vi "Arm Controller.vi"(8 "error in":errorcluster) -> ()   [LabVIEW 2017]
doc: "This VI executes continuously carrying out the current operation and responding to updates or new operations. It will often contain the timing or control code that is difficult to place directly in TeleOp. This VI generally opens all sensors and motors and isolates the rest of the robot code from knowing how the operations are carried out."
uses:
  <vilib>/Rock Robotics/WPI/Framework/Completion Status.ctl
  Arm Setpoints.ctl
  Arm Operations.ctl
  <vilib>/Rock Robotics/SystemInterfaces/DIO/FPGA_DIOPWMChannel.ctl
  <vilib>/Rock Robotics/SystemInterfaces/DIO/FPGA_DIOChannel.ctl
  <vilib>/Rock Robotics/WPI/Switch/WPI_SwitchOpenLimit.vi
  <vilib>/Rock Robotics/WPI/MotorControl/WPI_MotorControlOpen SPARK.vi
  Framework/Robot Global Data.vi
  <vilib>/Rock Robotics/Network Tables/NT Write Number.vi
panel:
  out "Lower Arm Limit Switch":bool
  out "Lift Arm Limit Switch":bool
  out "Switch Value":bool
  in  "Interactive Values":T1
  out "Current\nCmd":string
  in  "Buttons":cluster{"Execute Cmd":bool, "Abort Cmd":bool}
  out "Command Timing":cluster{"Start Time (ms)":u32, "Iterations":i32}
  out "Status":T3
  # "Tip: It may be helpful to observe inputs and sensor values.\nYou may also want to display tuning or debugging controls."
  # "Interactive Command: You may fill in the settings for a command\nand schedule it with the Execute button. You can observe and abort\nany command while fine tuning the code for the controller."
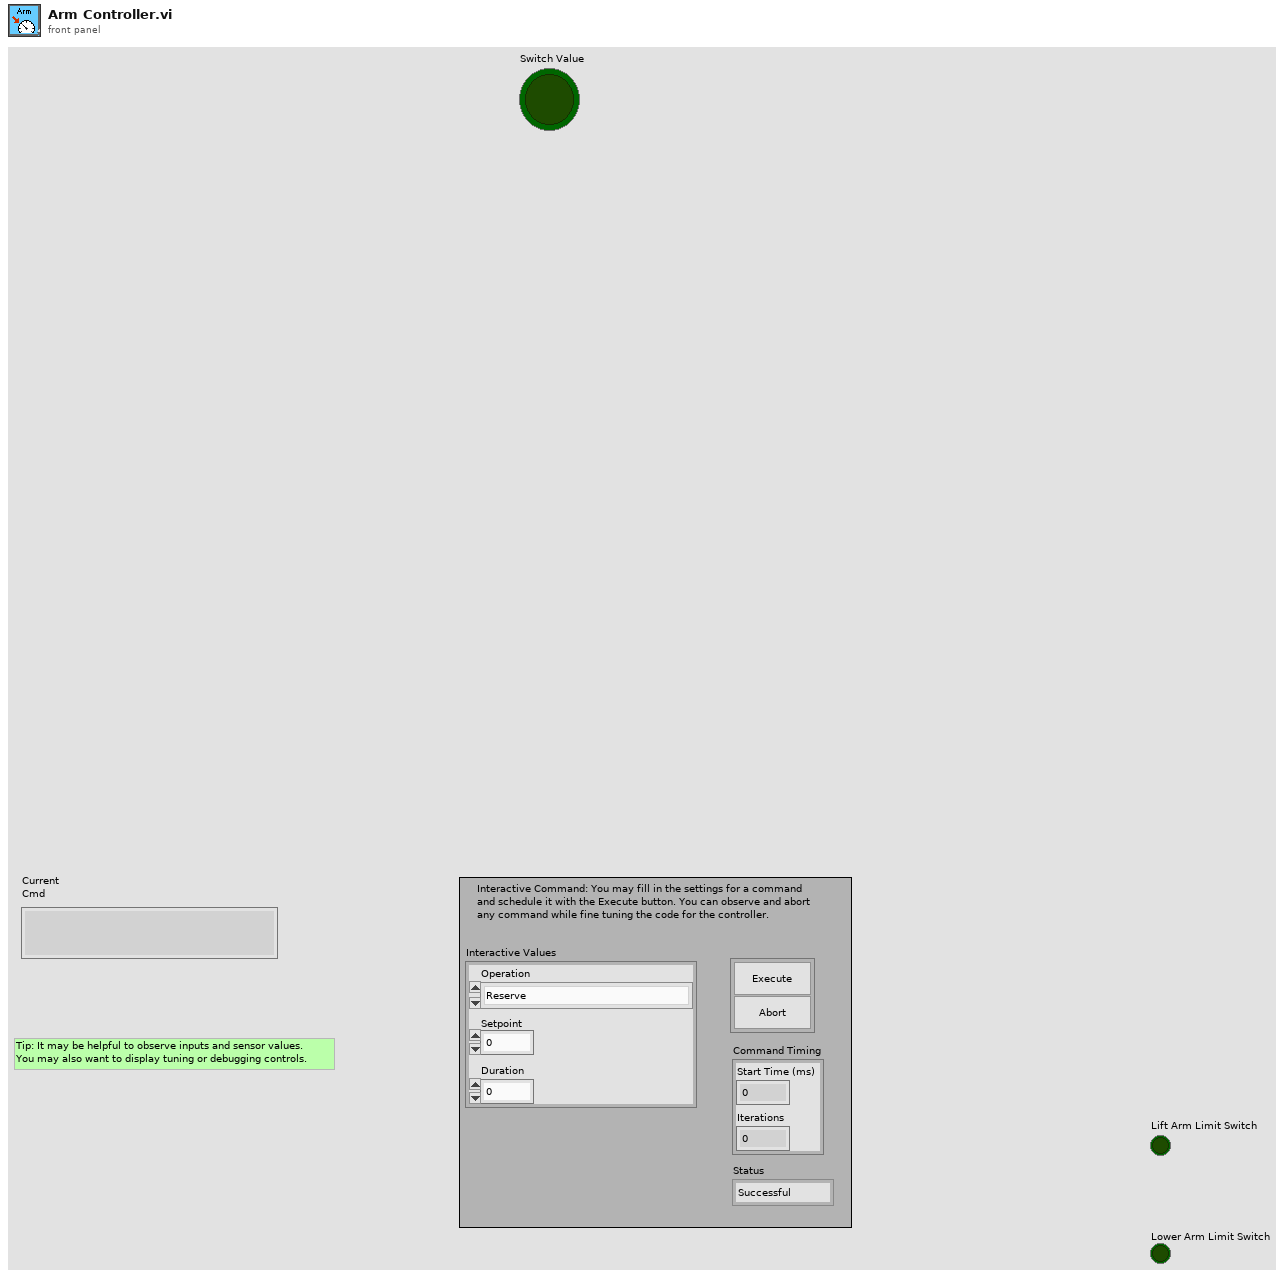
[diagram p1: front panel]
types:
  T1 = typedef "Arm Setpoints.ctl" = cluster{"Operation":T2, "Setpoint":dbl, "Duration":dbl}
  T2 = typedef "Arm Operations.ctl" = enum16{"Reserve", "Read Current", "Immediate", "Lift Arm", "Lower Arm ", "Button Lift Arm", "Button Lower Arm"}
  T3 = typedef "Completion Status.ctl" = enum16{"Successful", "Aborted", "Incomplete"}
  T4 = typedef "FPGA_DIOChannel.ctl" = enum8{"DIO 0", "DIO 1", "DIO 2", "DIO 3", "DIO 4", "DIO 5", "DIO 6", "DIO 7", "DIO 8", "DIO 9", "DIO MXP 0", "DIO MXP 1", "DIO MXP 2", "DIO MXP 3", "DIO MXP 4", "DIO MXP 5", "DIO MXP 6", "DIO MXP 7", "DIO MXP 8", "DIO MXP 9", "DIO MXP 10", "DIO MXP 11", "DIO MXP 12", "DIO MXP 13", "DIO MXP 14", "DIO MXP 15", "SPI Port CS1", "SPI Port CS2", "SPI Port CS3", "SPI Port MISO", "SPI Port MOSI", "Invalid"}
  T5 = typedef "FPGA_DIOPWMChannel.ctl" = enum8{"PWM 0", "PWM 1", "PWM 2", "PWM 3", "PWM 4", "PWM 5", "PWM 6", "PWM 7", "PWM 8", "PWM 9", "PWM MXP 0", "PWM MXP 1", "PWM MXP 2", "PWM MXP 3", "PWM MXP 4", "PWM MXP 5", "PWM MXP 6", "PWM MXP 7", "PWM MXP 8", "PWM MXP 9", "Invalid"}
  T6 = typedef "WPI_MotorControlDeviceRef.ctl" = cluster{"DeviceStatus":errorcluster, "Type":T7, "PWM":cluster{"PWM Channel":T5, "DeadBand":T8}, "CAN":cluster{"Device Number":u8, "SetOutput VI Ref":variant, "GetOutput VI Ref":variant, "Enable VI Ref":variant, "Disable VI Ref":variant, "Data":variant}, "Invert":bool, "DIO PWM":cluster{"PWM \"Enable\" Channel":T5, "DIOChannel":T4, "PWM Rate":dbl}}
  T7 = typedef "WPI_MotorControlType.ctl" = enum16{"PWM", "CAN", "DIO PWM"}
  T8 = typedef "WPI_PWMDeadband.ctl" = cluster{"Name":string, "maxPositivePwm":i32, "minPositivePwm":i32, "centerPwm":i32, "maxNegativePwm":i32, "minNegativePwm":i32, "angularRange":u16}
  T9 = typedef "WPI_SwitchDevRef.ctl" = cluster{"DevStatus":errorcluster, "DIO Channel":T4, "CntIndex":T10, "Normally Closed":bool}
  T10 = typedef "FPGA_CounterCtrSystemIndex.ctl" = enum8{"Ctr 0", "Ctr 1", "Ctr 2", "Ctr 3", "Ctr 4", "Ctr 5", "Ctr 6", "Ctr 7", "Invalid"}
  T11 = typedef "Command Status Info.ctl" = cluster{"Name":string, "Status":T3, "notifier out":T12}
  T12 = typedef "Completion Notifier.ctl" = refnum<notifier>
  T13 = cluster{"Current Command":T1, "Command Timing":cluster{"Start Time (ms)":u32, "Iterations":i32}, "Command Arguments":cluster{"Command Info":T11, "Description":string, "Default Command":T1, "queue out":refnum<queue>, "Subsystem Name":string}}
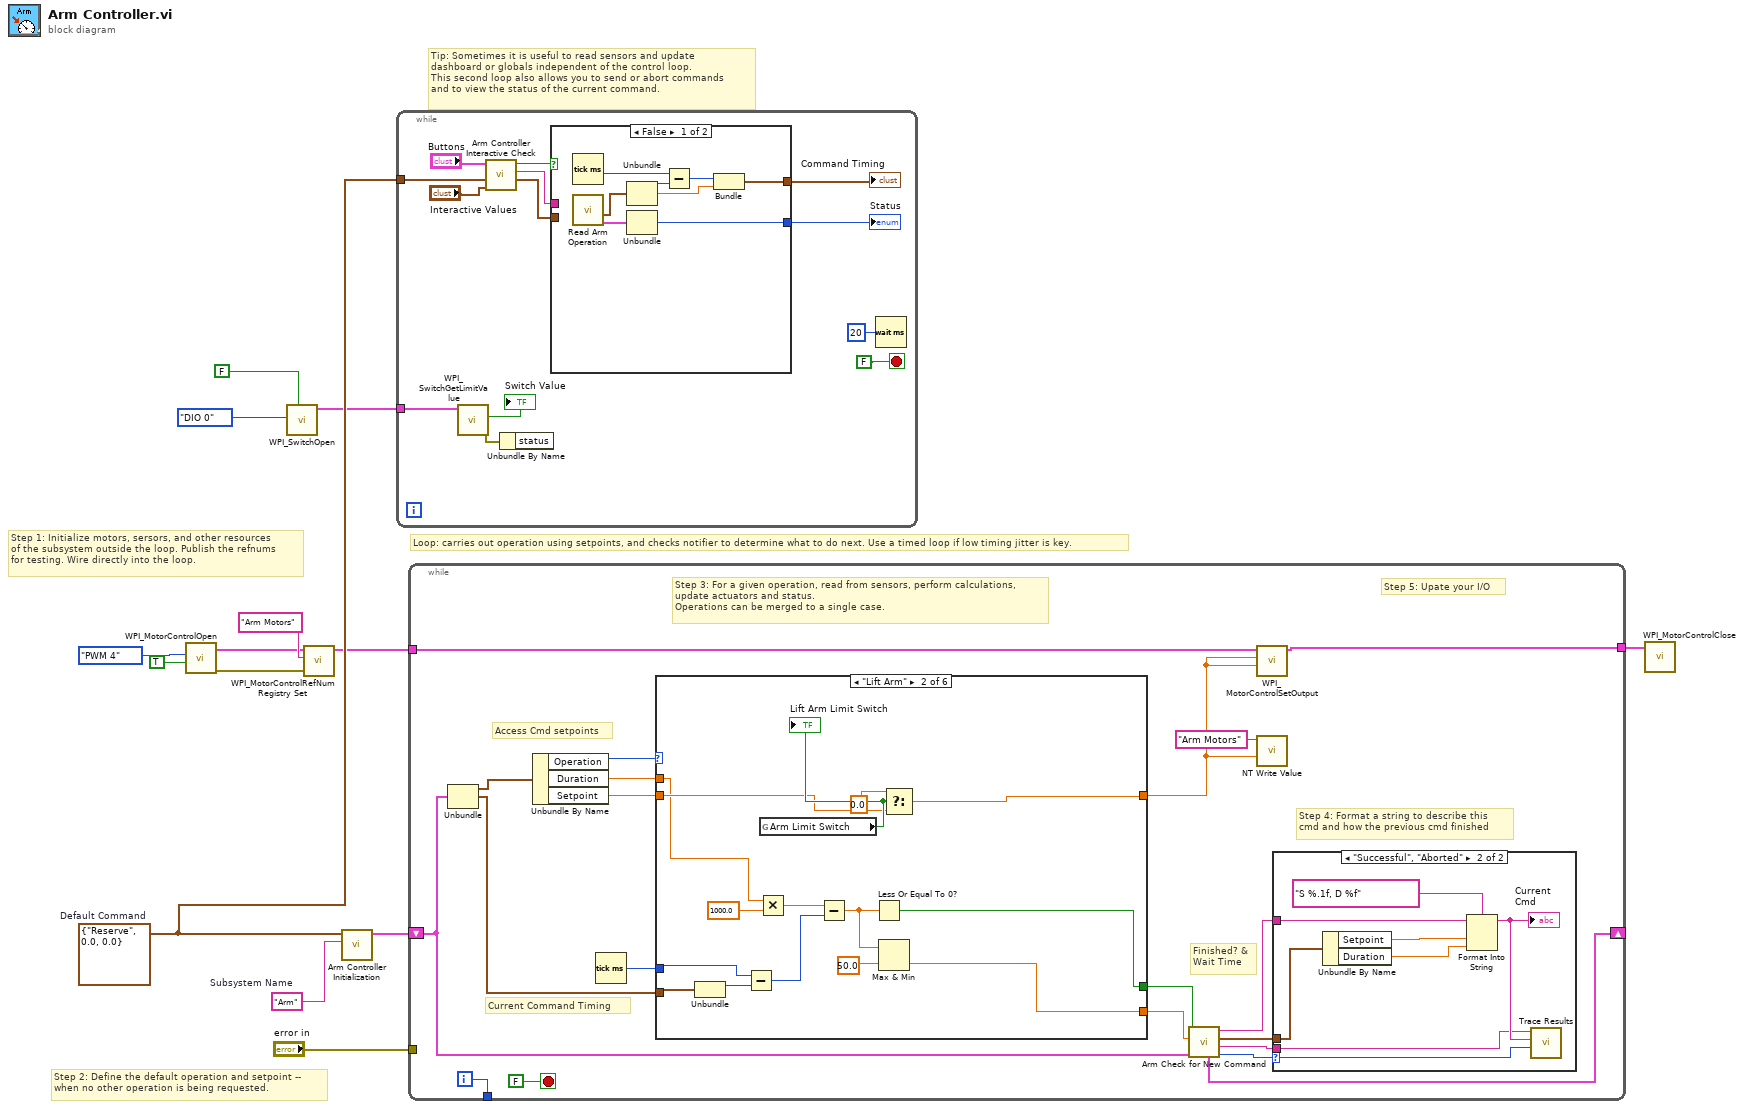
[diagram p0: block diagram]
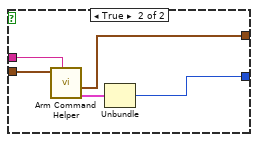
[diagram p2: hidden frame]
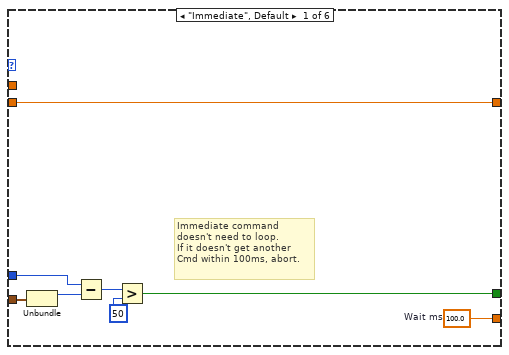
[diagram p4: hidden frame]
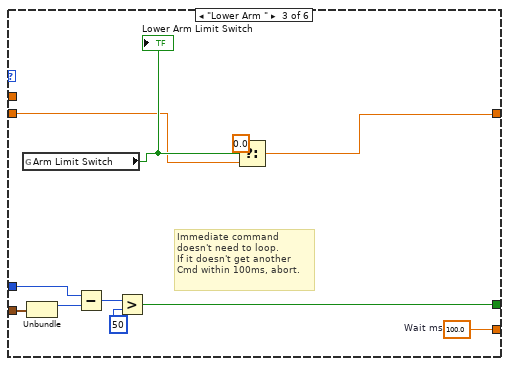
[diagram p5: hidden frame]
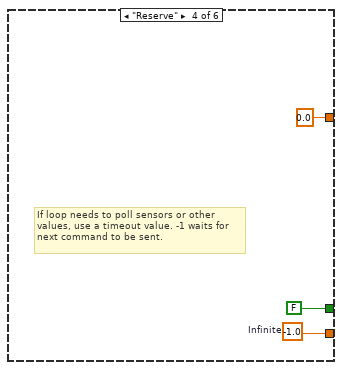
[diagram p6: hidden frame]
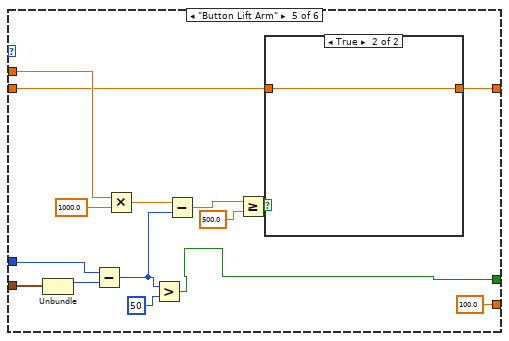
[diagram p7: hidden frame]
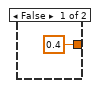
[diagram p8: hidden frame]
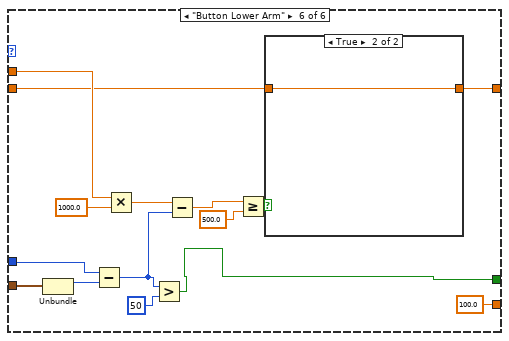
[diagram p9: hidden frame]
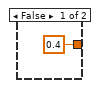
[diagram p10: hidden frame]
diagram:
  w11 = T1 {"Operation"=enum."Reserve", "Setpoint"=0.0, "Duration"=0.0}  # Default Command
  w12 = "Arm"  # Subsystem Name
  # "Tip: Sometimes it is useful to read sensors and update\ndashboard or globals independent of the control loop.\nThis second loop also allows you to send or abort commands\nand to view the status of the current command."
  # "Step 2: Define the default operation and setpoint --\nwhen no other operation is being requested."
  # "Step 1: Initialize motors, sersors, and other resources\nof the subsystem outside the loop. Publish the refnums\nfor testing. Wire directly into the loop."
  # "Loop: carries out operation using setpoints, and checks notifier to determine what to do next. Use a timed loop if low timing jitter is key."
  n1 = call-poly <vilib>:"WPI_MotorControlOpen.vi"("Eliminate Deadband"=TRUE, "PWM Channel"=FPGA_DIOPWMChannel."PWM 4") -> ("error out"=w3:errorcluster, "MotorControlDeviceRef"=w2:T6)  [unwired: 8 in]
  n2 = call-poly <vilib>:"WPI_SwitchOpen.vi"("Normally Closed"=FALSE, "DIO Channel"=FPGA_DIOChannel."DIO 0") -> ("SwitchDevRef"=w6:T9)  [unwired: 8 in, 1 out]
  n3 = call <vilib>:"WPI_MotorControlRefNum Registry Set.vi"("error in (no error)"=w3, "refnum name"="Arm Motors", "MotorControlDevRef"=w2) -> ("MotorControlDevRef"=w10:T6)  [unwired: 7 in, 1 out]
  n4 = call "Arm Controller Initialization.vi"("Subsystem Name"=w12, "Default Command"=w11) -> ("Current Command"=w13:T13)  [unwired: 9 in]
  n5 = while {
    tunnel: w11 -> [w24]
    tunnel: w6 -> [w15]
    stop <- FALSE stop-if-true
    n6 = call <vilib>:"WPI_SwitchGetLimitValue.vi"("SwitchDevRef"=w15) -> ("error out"=w16:errorcluster, "Switch Pressed"=→"Switch Value":bool)  [unwired: 8 in, 1 out]
    n7 = call "Arm Controller Interactive Check.vi"("Interactive Command in"="Interactive Values", "Default Command"=w24, "Buttons"="Buttons") -> ("Interactive Command out"=w21:T1, "Trace String"=w22:string, "Schedule"=w23:bool)  [unwired: 6 in]
    n8 = Unbundle By Name(w16) -> ()  [unwired: 1 out]
    n9 = case shown="False" w23 {
      tunnel: [w35 w40] -> w20
      tunnel: w21 -> [_ w38]
      tunnel: [w31 w36] -> w19
      tunnel: w22 -> [_ w39]
      frame False {
        n10 = Tick Count (ms)() -> (millisecond timer value=w30:u32)
        n11 = call "Read Arm Operation.vi"() -> ("Command Info"=w28:T11, "SubSystem Data"=w29:T1)  [unwired: 9 in, 1 out]
        n12 = Unbundle(w29) -> ("Operation"=w34:T2, "Setpoint"=w32:dbl)  [unwired: 1 out]
        n13 = Unbundle(w28) -> ("Status"=w35:T3)  [unwired: 2 out]
        n14 = Subtract(x=w30, y=w34) -> (x-y=w33:u32)
        n15 = Bundle(w33, "Setpoint"=w32) -> (w31:cluster{u32, "Setpoint":dbl})  [unwired: 1 in]
      }
      frame True {
        n16 = call "Arm Command Helper.vi"("Description"=w39, "SubSystem Data"=w38) -> ("Command Info Out"=w37:T11, "Command Timing"=w36:cluster{"Start Time (ms)":u32, "Iterations":i32})  [unwired: 7 in, 1 out]
        n17 = Unbundle(w37) -> ("Status"=w40:T3)  [unwired: 2 out]
      }
    }
    "Status" <- w20
    "Command Timing" <- w19
    n18 = Wait (ms)(milliseconds to wait=u32 20) -> ()  [unwired: 1 out]
  }
  n19 = while {
    shift-right: [w52] -> _
    shift-left: w13 -> [w41]
    tunnel: [w59] -> _
    tunnel: "error in" -> [_]
    tunnel: w10 -> [w42]
    tunnel: [w43] -> w1
    i -> [w59]
    stop <- FALSE stop-if-true
    # "Step 5: Upate your I/O"
    # "Step 4: Format a string to describe this\ncmd and how the previous cmd finished"
    # "Current Command Timing"
    # "Access Cmd setpoints"
    # "Finished? &\nWait Time"
    # "Step 3: For a given operation, read from sensors, perform calculations,\nupdate actuators and status.\nOperations can be merged to a single case."
    n20 = Unbundle(w41) -> ("Current Command"=w58:T1, "Command Timing"=w54:cluster{"Start Time (ms)":u32, "Iterations":i32})  [unwired: 1 out]
    n21 = Unbundle By Name(w58) -> ("Operation"=w57:T2, "Duration"=w56:dbl, "Setpoint"=w53:dbl)
    n22 = Tick Count (ms)() -> (millisecond timer value=w55:u32)
    n23 = case shown="\"Lift Arm\"" w57 {
      tunnel: [w76 w79 w102 w105 100.0 ("Infinite") 100.0 ("Infinite")] -> w46
      tunnel: [w70 w78 w96 FALSE ("ignore previous (F)") w107 w124] -> w47
      tunnel: w54 -> [w72 w80 w98 _ w116 w133]
      tunnel: w56 -> [_ w77 _ _ w115 w132]
      tunnel: w55 -> [w71 w81 w97 _ w117 w134]
      tunnel: w53 -> [w69 w89 w93 _ w111 w128]
      tunnel: [w69 w88 w92 0.0 ("Angle") w110 w127] -> w44
      frame "Immediate", Default {
        w76 = 100.0  # Wait ms
        # "Immediate command\ndoesn't need to loop.\nIf it doesn't get another\nCmd within 100ms, abort."
        n24 = Unbundle(w72) -> ("Start Time (ms)"=w75:u32)  [unwired: 1 out]
        n25 = Subtract(x=w71, y=w75) -> (x-y=w74:u32)
        n26 = Greater?(x=w74, y=u8 50 ("Left Motor")) -> (0:w70:bool)
      }
      frame "Lift Arm" {
        n27 = Unbundle(w80) -> ("Start Time (ms)"=w84:u32)  [unwired: 1 out]
        n28 = Subtract(x=w81, y=w84) -> (x-y=w87:u32)
        n29 = Multiply(x=w77, y=1000.0) -> (x*y=w86:dbl)
        n30 = global read "Robot Global Data.vi" "Arm Limit Switch"() -> (w90:bool)
        "Lift Arm Limit Switch" <- w90
        n31 = Subtract(x=w86, y=w87) -> (x-y=w83:dbl)
        n32 = Less Or Equal To 0?(x=w83) -> (x <= 0?=w78:bool)
        n33 = Max & Min(x=w83, y=50.0) -> (min(x,y)=w79:dbl)  [unwired: 1 out]
        n34 = Select(t=0.0, s=w90, f=w89) -> (s? t:f=w88:dbl)
      }
      frame "Lower Arm " {
        w102 = 100.0  # Wait ms
        # "Immediate command\ndoesn't need to loop.\nIf it doesn't get another\nCmd within 100ms, abort."
        n35 = global read "Robot Global Data.vi" "Arm Limit Switch"() -> (w94:bool)
        "Lower Arm Limit Switch" <- w94
        n36 = Unbundle(w98) -> ("Start Time (ms)"=w101:u32)  [unwired: 1 out]
        n37 = Subtract(x=w97, y=w101) -> (x-y=w100:u32)
        n38 = Greater?(x=w100, y=u8 50 ("Left Motor")) -> (0:w96:bool)
        n39 = Select(t=0.0, s=w94, f=w93) -> (s? t:f=w92:dbl)
      }
      frame "Reserve" {
        w105 = -1.0  # Infinite
        # "If loop needs to poll sensors or other\nvalues, use a timeout value. -1 waits for\nnext command to be sent."
      }
      frame "Button Lift Arm" {
        n40 = Unbundle(w116) -> ("Start Time (ms)"=w118:u32)  [unwired: 1 out]
        n41 = Subtract(x=w117, y=w118) -> (x-y=w109:u32)
        n42 = Multiply(x=w115, y=1000.0) -> (x*y=w120:dbl)
        n43 = Greater?(x=w109, y=u8 50 ("Left Motor")) -> (0:w107:bool)
        n44 = Subtract(x=w120, y=w109) -> (x-y=w114:dbl)
        n45 = Greater Or Equal?(x=w114, y=500.0 ("x")) -> (x >= y?=w112:bool)
        n46 = case shown="True" w112 {
          tunnel: w111 -> [_ w122]
          tunnel: [0.4 ("Setpoint") w122] -> w110
          frame False {
          }
          frame True {
          }
        }
      }
      frame "Button Lower Arm" {
        n47 = Unbundle(w133) -> ("Start Time (ms)"=w135:u32)  [unwired: 1 out]
        n48 = Subtract(x=w134, y=w135) -> (x-y=w126:u32)
        n49 = Multiply(x=w132, y=1000.0) -> (x*y=w137:dbl)
        n50 = Greater?(x=w126, y=u8 50 ("Left Motor")) -> (0:w124:bool)
        n51 = Subtract(x=w137, y=w126) -> (x-y=w131:dbl)
        n52 = Greater Or Equal?(x=w131, y=500.0 ("x")) -> (x >= y?=w129:bool)
        n53 = case shown="True" w129 {
          tunnel: w128 -> [_ w139]
          tunnel: [0.4 ("Setpoint") w139] -> w127
          frame False {
          }
          frame True {
          }
        }
      }
    }
    n54 = call "Arm Check for New Command.vi"("Current Command"=w41, "Wait time (ms)"=w46, "Finished?"=w47) -> ("Completion"=w48:T3, "Subsystem Name"=w49:string, "Current Command"=w50:T1, "Initial Trace String"=w51:string, "NextCommand"=w52:T13)  [unwired: 4 in]
    n55 = call <vilib>:"WPI_MotorControlSetOutput.vi"("options"=w44, "Output"=w44, "MotorControlDevRef"=w42) -> ("MotorControlDevRef"=w43:T6)  [unwired: 6 in, 2 out]
    n56 = call-poly <vilib>:"NT Write Value.vi"("Numeric"=w44, "Name"="Arm Motors") -> ()  [unwired: 9 in, 1 out]
    n57 = case shown="\"Successful\", \"Aborted\"" w48 {
      selector: w48 -> [_ w68]
      tunnel: w51 -> [_ w64]
      tunnel: w50 -> [_ w65]
      tunnel: w49 -> [_ w61]
      frame "Incomplete", Default {
        # "Continuing current command"
      }
      frame "Successful", "Aborted" {
        # "Report and setup for next command"
        n58 = Unbundle By Name(w65) -> ("Setpoint"=w67:dbl, "Duration"=w62:dbl)
        n59 = Format Into String(format string="S %.1f, D %f", initial string=w64, w67, w62) -> (resulting string=w63:string)  [unwired: 1 in, 1 out]
        "Current\nCmd" <- w63
        n60 = call <vilib>:"Trace Results.vi"("Status of previous command"=w68, "Description"=w63, "Subsystem"=w61) -> ()  [unwired: 9 in]
      }
    }
  }
  n61 = call <vilib>:"WPI_MotorControlClose.vi"("MotorControlDevRef"=w1) -> ()  [unwired: 10 in, 1 out]
